vi "Copy From IMAQ.vi"() -> ()   [LabVIEW 2020]
uses:
  LabVIEW/g_ar_toolkit.common/Image Size (Integer).ctl
  LabVIEW/g_ar_toolkit.image/Raw Memory Information.ctl
  LabVIEW/g_ar_toolkit.image/Raw Memory Information Dimension.ctl
  LabVIEW/g_ar_toolkit.image/NewImageARGB.vi
  LabVIEW/g_ar_toolkit.image/NewImageARGB.vi/3321fa97-f432-4e1e-8db9-a0df79aed21b.vi
  LabVIEW/g_ar_toolkit.image/ARGB Colour to U32 Pixel Value.vi
  LabVIEW/g_ar_toolkit.image/CopyRawMemoryToImageARGB.vi/e0109ec8-11ee-4a07-aeee-d632e4e22c38.vi
  LabVIEW/g_ar_toolkit.image/DrawImageToPictureARGB.vi/8cd07b1b-062e-4fe4-9e87-2eb3dc89fe0e.vi
  LabVIEW/g_ar_toolkit.common/Module Path.vi
  <vilib>/Utility/error.llb/Error Cluster From Error Code.vi
  LabVIEW/g_ar_toolkit.image/NewImageARGBArray.vi
  <vilib>/vision/EDVR.llb/IMAQ ImageToEDVR 2D U32.vi
  LabVIEW/g_ar_toolkit.image/DrawImageToPictureARGB.vi
  LabVIEW/g_ar_toolkit.image/CopyRawMemoryToImageARGB.vi
  LabVIEW/g_ar_toolkit.image/g_ar_toolkit.image.lvlib
  LabVIEW/g_ar_toolkit.common/g_ar_toolkit.common.lvlib
panel:
  in  "Mode":T1(ring)
  out "IMAQ":T2(plugin-control)
  out "Ouput":picture
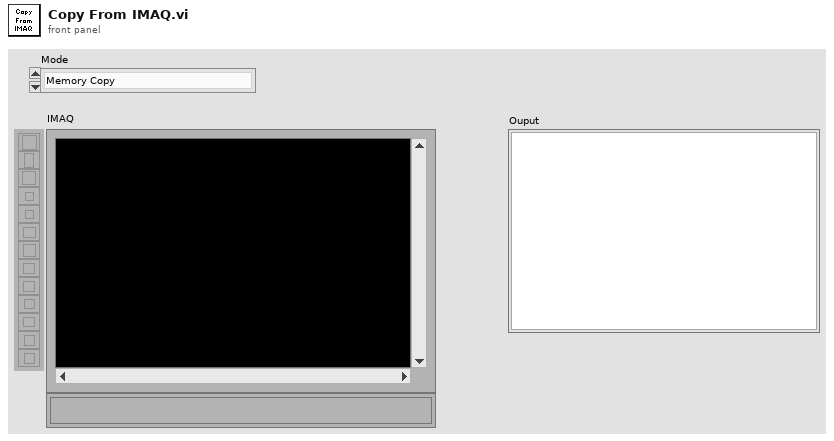
[diagram p1: front panel]
types:
  T1 = enum16{"Memory Copy", "EDVR Access", "Array Values"}
  T2 = typedef "IMAQ Image.ctl" = refnum<image>
  T3 = typedef "Image Type" = u32
  T4 = typedef "g_ar_toolkit.common.lvlib/Image Size (Integer).ctl" = cluster{"Width":u16, "Height":u16}
  T5 = enum32{"Map Pixel Pointer", "Unmap Pixel Pointer", "Get Pixels Infos"}
  T6 = typedef "g_ar_toolkit.image.lvlib/Raw Memory Information.ctl" = cluster{"Memory Address":u64, "Dimension 0":T7, "Dimension 1":T7}
  T7 = typedef "g_ar_toolkit.image.lvlib/Raw Memory Information Dimension.ctl" = cluster{"Size":u16, "Stride":u32}
  T8 = typedef "g_ar_toolkit.image.lvlib/ARGB Image.ctl" = refnum<data-value>
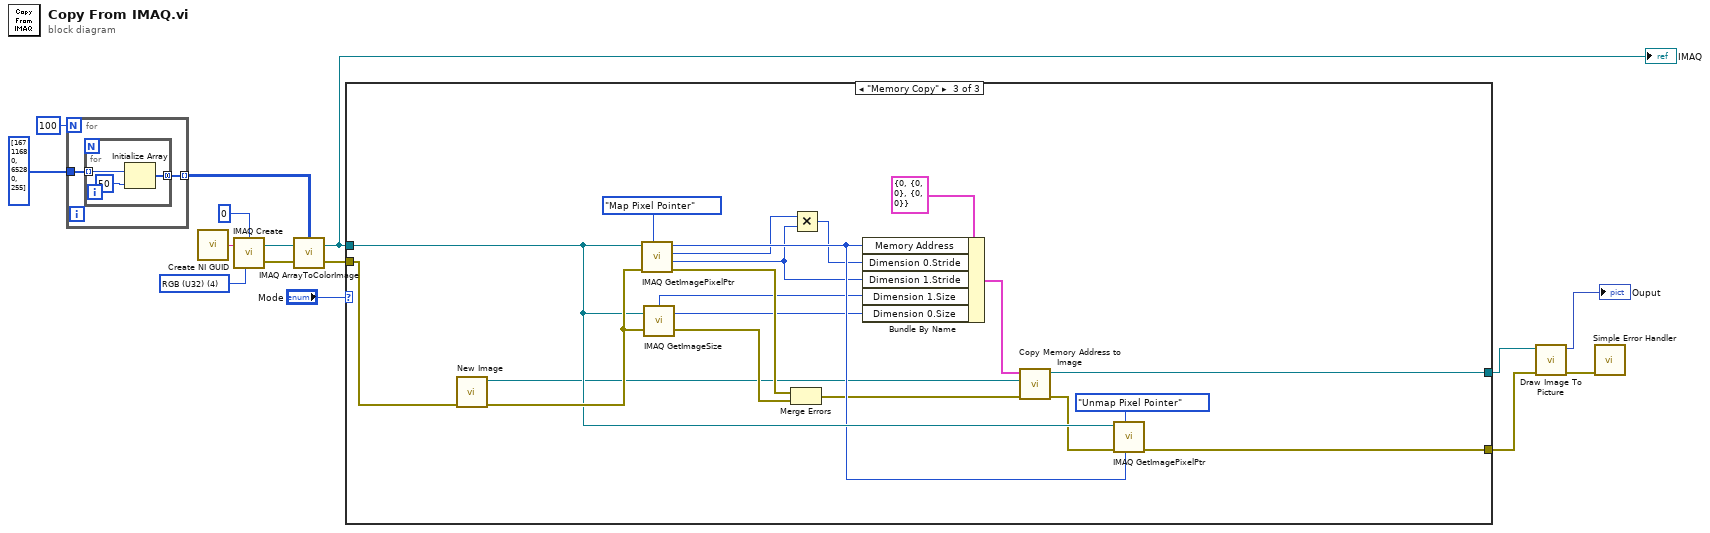
[diagram p0: block diagram]
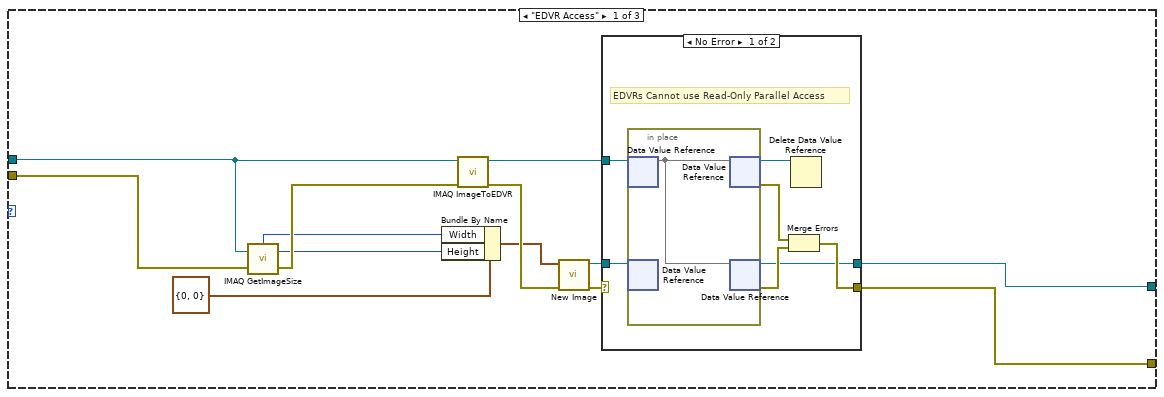
[diagram p2: hidden frame]
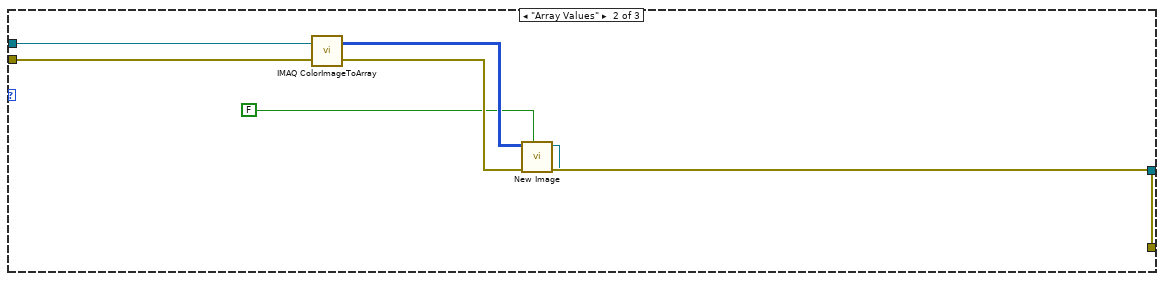
[diagram p4: hidden frame]
diagram:
  w11 = T3 4 items=["Grayscale (U8)", "Grayscale (I16)", "Grayscale (SGL)", "Complex (CSG)", "RGB (U32)", "HSL (U32)", "RGB (U64)", "Grayscale (U16)"] ("Image Type")
  n1 = for {
    N: 100 -> [_]
    tunnel: u32[] [16711680, 65280, 255] ("color(black)") -> [w17]
    tunnel: [w16] -> w12 mode=indexing
    n2 = for {
      tunnel: w17 -> [w20] mode=indexing
      tunnel: [w18] -> w16 mode=concatenating
      n3 = Initialize Array(w20, 50 ("dimension size")) -> (w18:u32[])
    }
  }
  n4 = call <vilib>:"Create NI GUID.vi"() -> ("NI GUID"=w2:string)
  n5 = call "IMAQ Create"("Border Size"=0, "Image Name"=w2, "Image Type"=w11) -> ("New Image"=w15:T2, "error out"=w7:errorcluster)  [unwired: 2 in]
  n6 = call "IMAQ ArrayToColorImage"("Image Pixels (U32)"=w12, "Image"=w15, "error in (no error)"=w7) -> ("Image Out"=w8:T2, "error out"=w10:errorcluster)  [unwired: 2 in]
  "IMAQ" <- w8
  n7 = case shown="\"Memory Copy\"" "Mode" {
    tunnel: w10 -> [w24 w48 w68]
    tunnel: w8 -> [w23 w49 w67]
    tunnel: [w21 w46 w66] -> w6
    tunnel: [w22 w45 w65] -> w5
    frame "EDVR Access" {
      n8 = call "IMAQ GetImageSize"("Image"=w23, "error in (no error)"=w24) -> ("Y Resolution"=w29:i32, "X Resolution"=w28:i32, "error out"=w32:errorcluster)  [unwired: 2 in]
      n9 = Bundle By Name(cluster=T4 {"Width"=0, "Height"=0} ("Preallocated Image Size (Default: 0,0)"), "Width"=w28, "Height"=w29) -> (w30:T4)
      n10 = call-poly <vilib>:"IMAQ ImageToEDVR.vi"("error out"=w32, "Image"=w23) -> ("error out"=w33:errorcluster, "EDVR 2D U32"=w26:refnum<data-value>)  [unwired: 7 in, 1 out]
      n11 = call-poly "New Image.vi"("error in (no error)"=w33, "Preallocated Image Size (Default: 0,0)"=w30) -> ("error out"=w25:errorcluster, "New ARGB Image"=w27:T8)  [unwired: 8 in]
      n12 = case shown="No Error" w25 {
        selector: w25 -> [_ w43]
        tunnel: w27 -> [w40 w42]
        tunnel: w26 -> [w39 _]
        tunnel: [w36 w43] -> w21
        tunnel: [w35 w42] -> w22
        frame No Error {
          # "EDVRs Cannot use Read-Only Parallel Access"
          n13 = in-place {
            n14 = in-place-dvr #1(w39) -> (w41:u32[][])  [unwired: 1 out]
            n15 = in-place-dvr #2(w40) -> ()  [unwired: 2 out]
            n16 = in-place-dvr #1(w41) -> (w34:refnum<data-value>, w37:errorcluster)
            n17 = in-place-dvr #2(w41) -> (w35:T8, w38:errorcluster)
          }
          n18 = Merge Errors(w37, w38) -> (w36:errorcluster)
          n19 = Delete Data Value Reference(data value reference=w34) -> ()  [unwired: 1 in, 2 out]
        }
        frame Error {
        }
      }
    }
    frame "Array Values" {
      n20 = call "IMAQ ColorImageToArray"("Image"=w49, "error in (no error)"=w48) -> ("Image Pixels (U32)"=w47:u32[][], "error out"=w50:errorcluster)  [unwired: 2 in, 1 out]
      n21 = call-poly "New Image.vi"("Set Alpha Values to 255 (Default: True)"=FALSE, "error in (no error)"=w50, "U32 ARBG Data  (Default: Empty)"=w47) -> ("error out"=w46:errorcluster, "New ARGB Image"=w45:T8)  [unwired: 7 in]
    }
    frame "Memory Copy" {
      n22 = call-poly "New Image.vi"("error in (no error)"=w68) -> ("error out"=w70:errorcluster, "New ARGB Image"=w52:T8)  [unwired: 9 in]
      n23 = call "IMAQ GetImagePixelPtr"("Function"=T5."Map Pixel Pointer", "error in (no error)"=w70, "Image"=w67) -> ("error out"=w63:errorcluster, "Pixel Size (Bytes)"=w57:i32, "LineWidth(Pixels)"=w59:i32, "Pixel Pointer out"=w64:u64)  [unwired: 3 in, 2 out]
      n24 = call "IMAQ GetImageSize"("Image"=w67, "error in (no error)"=w70) -> ("Y Resolution"=w55:i32, "X Resolution"=w56:i32, "error out"=w69:errorcluster)  [unwired: 2 in]
      n25 = Merge Errors(w63, w69) -> (w51:errorcluster)
      n26 = Multiply(x=w59, y=w57) -> (x*y=w58:i32)
      n27 = Bundle By Name(cluster=T6 {"Memory Address"=0, "Dimension 0"={"Size"=0, "Stride"=0}, "Dimension 1"={"Size"=0, "Stride"=0}} ("Source"), "Memory Address"=w64, "Dimension 0.Stride"=w58, "Dimension 1.Stride"=w57, "Dimension 1.Size"=w56, "Dimension 0.Size"=w55) -> (w60:T6)
      n28 = call-poly "Copy Memory Address to Image.vi"("error in (no error)"=w51, "ARGB Image Destination"=w52, "Source"=w60) -> ("error out"=w54:errorcluster, "ARGB Image Destination (Duplicate)"=w65:T8)  [unwired: 7 in]
      n29 = call "IMAQ GetImagePixelPtr"("Pixel Pointer in"=w64, "Function"=T5."Unmap Pixel Pointer", "error in (no error)"=w54, "Image"=w67) -> ("error out"=w66:errorcluster)  [unwired: 2 in, 5 out]
    }
  }
  n30 = call-poly "Draw Image To Picture.vi"("error in (no error)"=w6, "ARGB Image Source"=w5) -> ("error out"=w3:errorcluster, "Picture"=→"Ouput":picture)  [unwired: 8 in]
  n31 = call <vilib>:"Simple Error Handler.vi"("error in (no error)"=w3) -> ()  [unwired: 4 in, 5 out]
